vi "NF WF1973_74 SWE Spac.vi"(6 "Read(F)":bool, 8 "error in (no error)":errorcluster caption="Error IN", 9 "Spacing(Liner)":u16(ring) items=["Liner", "Logarithmic"], 10 "Ch(Ch1)":bool, 11 "VISAsession":refnum<visa-resource-name>) -> (0 "error out":errorcluster caption="Error OUT", 2 "Query Spacing":string, 3 "CopyVISAsession":refnum<visa-resource-name>)   [LabVIEW 2010]
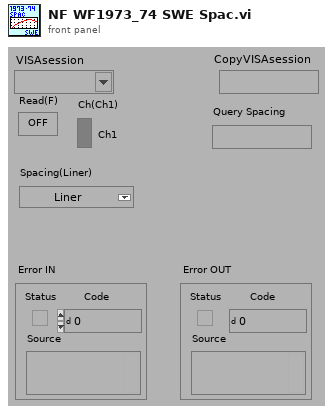
[diagram p1: front panel]
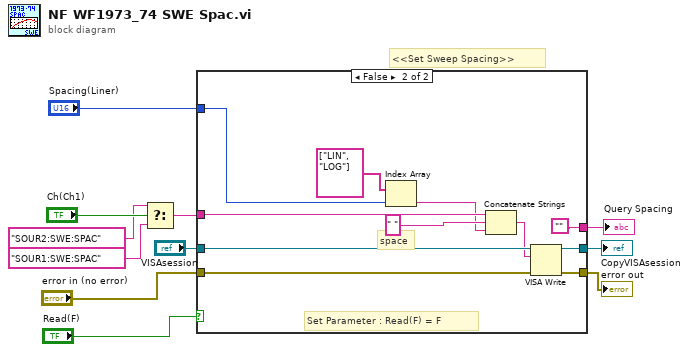
[diagram p0: block diagram]
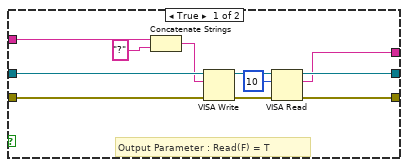
[diagram p2: hidden frame]
diagram:
  # "<<Set Sweep Spacing>>"
  n1 = Select(t="SOUR2:SWE:SPAC" ("文字列"), s="Ch(Ch1)", f="SOUR1:SWE:SPAC" ("文字列")) -> (s? t:f=w4:string)
  n2 = case shown="FALSE" "Read(F)" {
    tunnel: "VISAsession" -> [w22 w33]
    tunnel: [w19 w31] -> w10
    tunnel: [w18 w32] -> w9
    tunnel: "error in (no error)" -> [w17 w27]
    tunnel: w4 -> [w15 w28]
    tunnel: [w12 ""] -> w6
    tunnel: "Spacing(Liner)" -> [_ w25]
    frame True {
      # "Output Parameter : Read(F) = T"
      n3 = Concatenate Strings(w15, "?" ("形式文字列")) -> (w13:string)
      n4 = VISA Write(VISA resource name=w22, write buffer=w13, error in (no error)=w17) -> (VISA resource name out=w20:refnum<visa-resource-name>, error out=w21:errorcluster)  [unwired: 1 out]
      n5 = VISA Read(VISA resource name=w20, byte count=u32 10 ("バイトカウント（0）"), error in (no error)=w21) -> (VISA resource name out=w19:refnum<visa-resource-name>, read buffer=w12:string, error out=w18:errorcluster)  [unwired: 1 out]
    }
    frame False {
      # "space"
      # "Set Parameter : Read(F) = F"
      n6 = Index Array(array=string[] ["LIN", "LOG"] ("配列"), index=w25) -> (element=w26:string)
      n7 = Concatenate Strings(w28, " ", w26) -> (w30:string)
      n8 = VISA Write(VISA resource name=w33, write buffer=w30, error in (no error)=w27) -> (VISA resource name out=w31:refnum<visa-resource-name>, error out=w32:errorcluster)  [unwired: 1 out]
    }
  }
  "error out" <- w9
  "CopyVISAsession" <- w10
  "Query Spacing" <- w6
